vi "GetTestResult.vi"(11 "GuiRef":T1={"StringOut"=refnum, "AbortOnFail"=refnum, "SN"=refnum, "SN_Length"=refnum, "TestResult"=refnum, "CycleTime"=refnum, "ErrorCode"=refnum, "UUTStatus"=refnum, "DataBaseEnable?"=refnum, "DUTModel"=refnum, "FixtureID"=refnum, "OperatorID"=refnum, "SNReady"=refnum, "StopSlot"=refnum, "NextStep"=refnum, "PassYeild"=refnum, "Failed"=refnum, "Passed"=refnum, "Tested"=refnum, "TestItemsCtl"={"StepName"="", "TestEnable"=FALSE, "LoopCount"=0, "StopOnFail"=FALSE, "Index"=0, "TestName"="", "通道"="", "参数"="", "TimeStart"=0}, "ProcessBar"=refnum, "Slot"=enum."Slot1", "Row"=3, "States"=refnum, "TestMode"=refnum, "循环次数-DUT"=refnum, "波形图"=refnum, "产品型号"=refnum, "子面板"=refnum, "测试失败项目"=refnum, "测试结果"=refnum, "DUT"=refnum, "Starttime"=refnum, "SlotReady"=refnum, "版本信息"=refnum, "WIFI_1"=refnum, "WIFI_2"=refnum, "直通率"=refnum, "卡1开卡结果"=refnum, "卡2开卡结果"=refnum}) -> (1 "FailStep":string, 2 "PASS/FAIL":bool)   [LabVIEW 2013]
uses:
  SysControl/Reference.ctl
  SysControl/TestItemsCTL.ctl
  SysControl/Slot.ctl
  SysControl/LEDState.ctl
panel:
  out "FAIL项目":string
  out "PASS项目":string
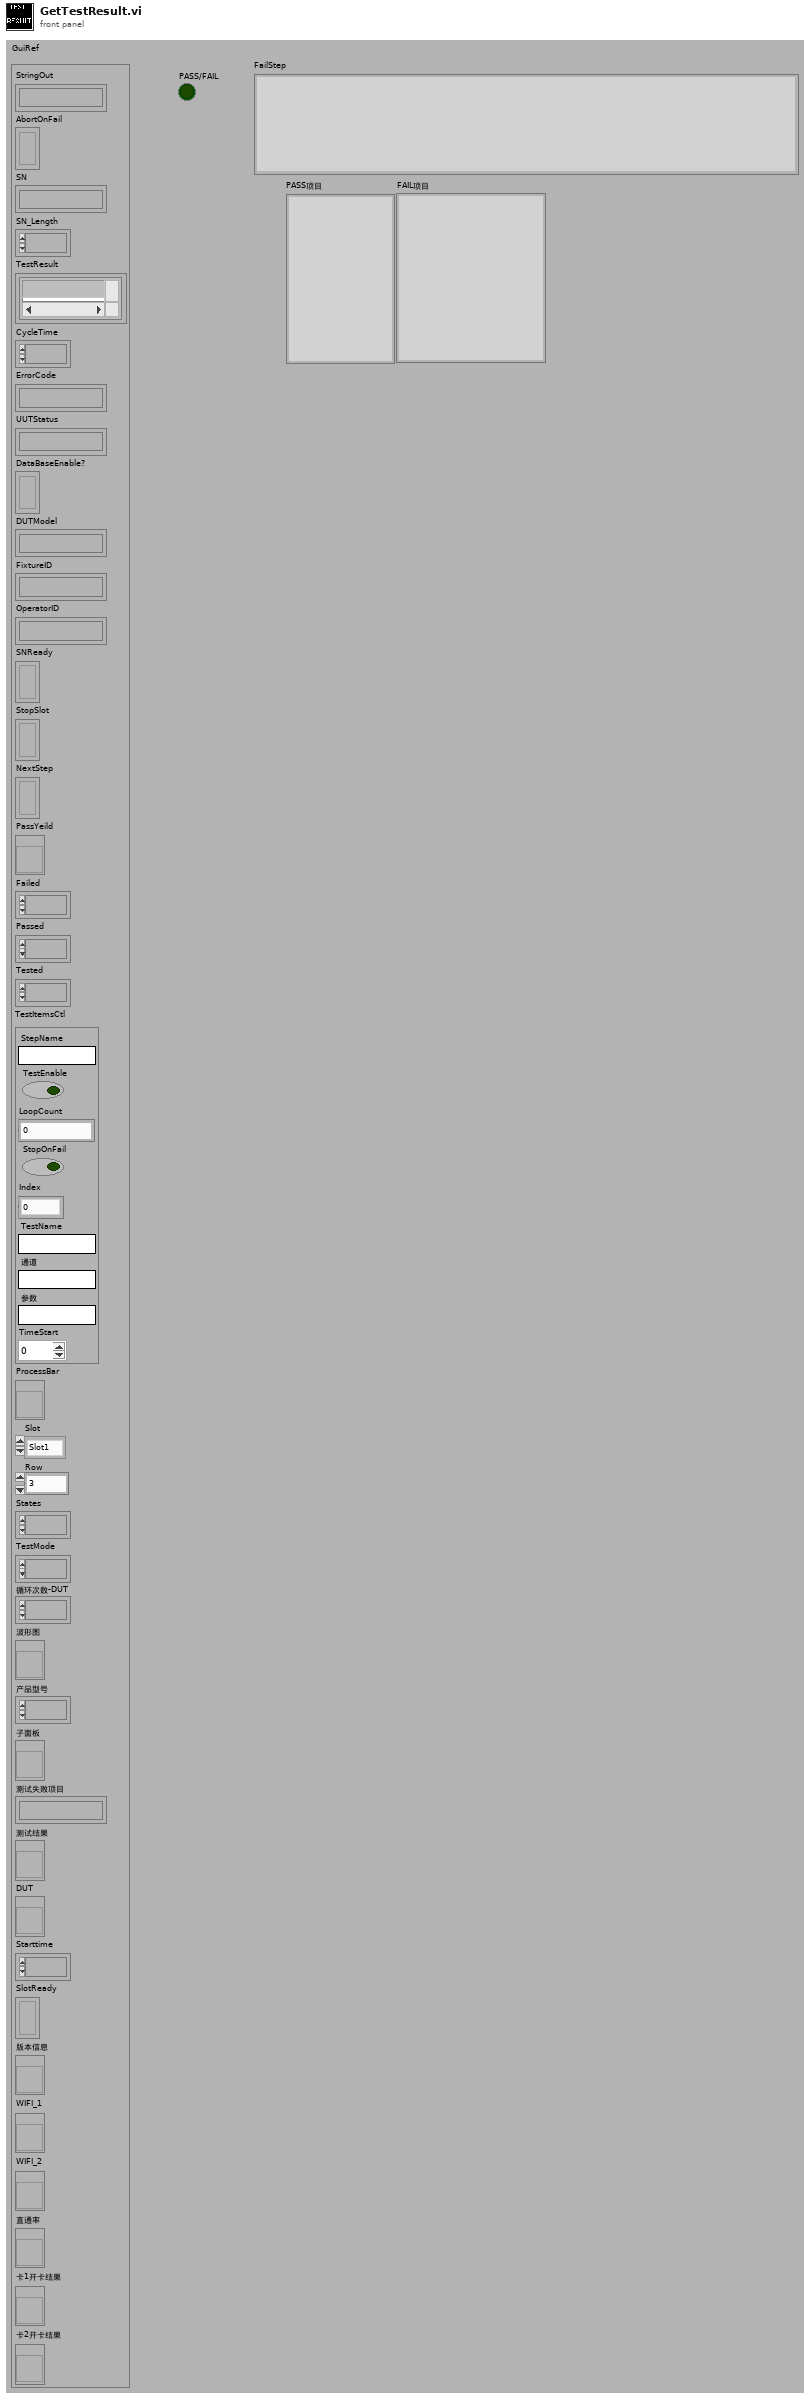
[diagram p1: front panel]
types:
  T1 = typedef "Reference.ctl" = cluster{"StringOut":refnum<vi>, "AbortOnFail":refnum<vi>, "SN":refnum<vi>, "SN_Length":refnum<vi>, "TestResult":refnum<vi>, "CycleTime":refnum<vi>, "ErrorCode":refnum<vi>, "UUTStatus":refnum<vi>, "DataBaseEnable?":refnum<vi>, "DUTModel":refnum<vi>, "FixtureID":refnum<vi>, "OperatorID":refnum<vi>, "SNReady":refnum<vi>, "StopSlot":refnum<vi>, "NextStep":refnum<vi>, "PassYeild":refnum<vi>, "Failed":refnum<vi>, "Passed":refnum<vi>, "Tested":refnum<vi>, "TestItemsCtl":T2, "ProcessBar":refnum<vi>, "Slot":T3, "Row":u32, "States":refnum<vi>, "TestMode":refnum<vi>, "循环次数-DUT":refnum<vi>, "波形图":refnum<vi>, "产品型号":refnum<vi>, "子面板":refnum<vi>, "测试失败项目":refnum<vi>, "测试结果":refnum<vi>, "DUT":refnum<vi>, "Starttime":refnum<vi>, "SlotReady":refnum<vi>, "版本信息":refnum<vi>, "WIFI_1":refnum<vi>, "WIFI_2":refnum<vi>, "直通率":refnum<vi>, "卡1开卡结果":refnum<vi>, "卡2开卡结果":refnum<vi>}
  T2 = typedef "TestItemsCTL.ctl" = cluster{"StepName":string, "TestEnable":bool, "LoopCount":i32, "StopOnFail":bool, "Index":u32, "TestName":string, "通道":string, "参数":string, "TimeStart":u32}
  T3 = typedef "Slot.ctl" = enum16{"Slot1", "Slot2", "Slot3", "Slot4"}
  T4 = typedef "LEDState.ctl" = enum16{"默认", "闪烁", "停止闪烁", "真", "假"}
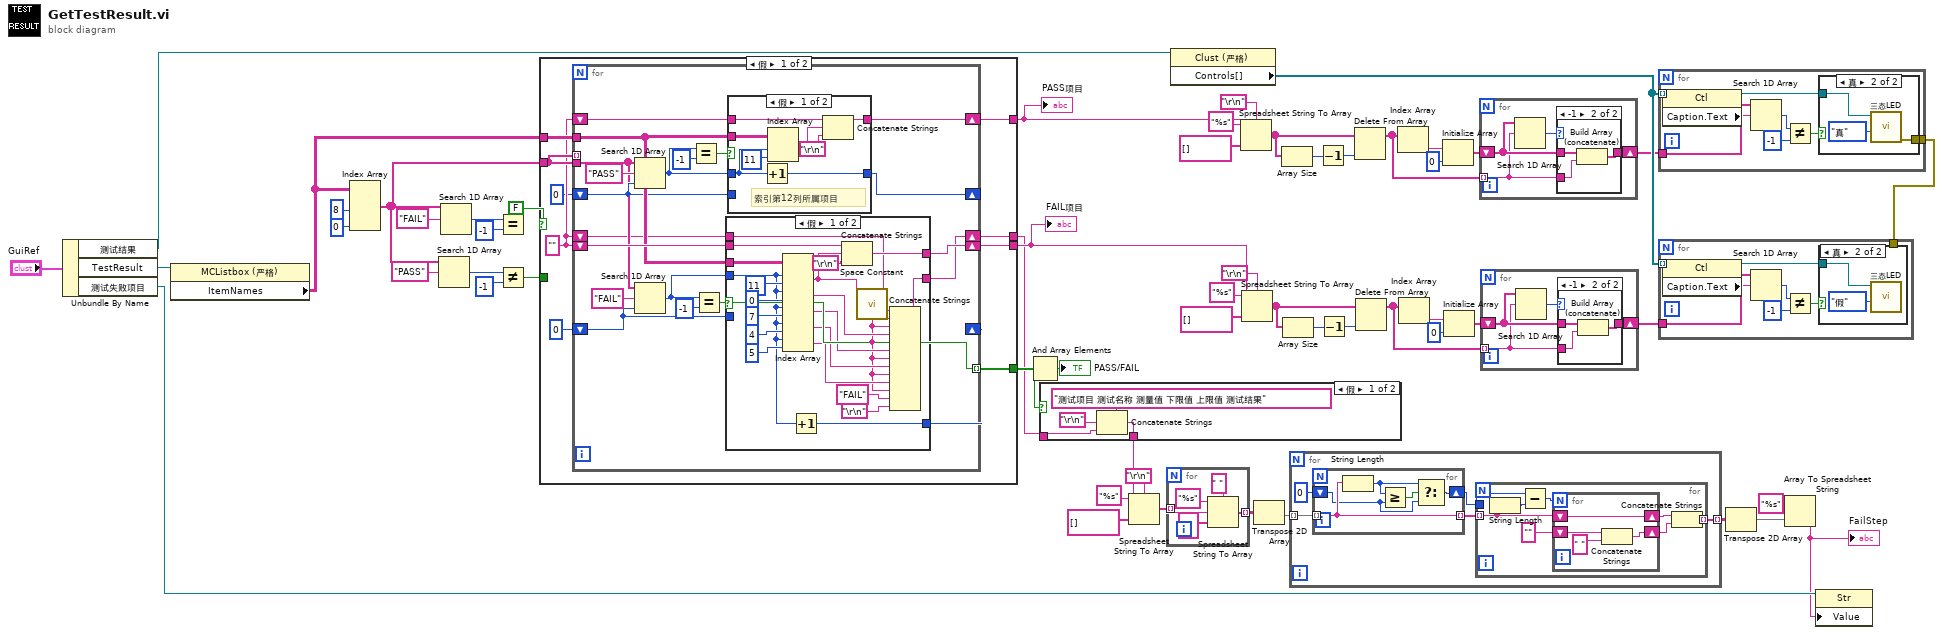
[diagram p0: block diagram]
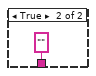
[diagram p2: hidden frame]
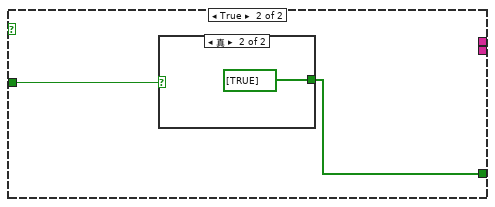
[diagram p9: hidden frame]
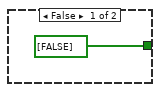
[diagram p10: hidden frame]
diagram:
  n1 = Unbundle By Name("GuiRef") -> ("测试结果"=w39:refnum<vi>, "TestResult"=w44:refnum<vi>, "测试失败项目"=w15:refnum<vi>)
  n2 = property class="MCListbox (严格)"(reference=w44) -> ("ItemNames"=w43:string[][])  [unwired: 1 in, 2 out]
  n3 = Index Array(array=w43, index (col) #1=8 ("禁用的索引 (列)"), index (col) #2=0 ("index (col)")) -> (element #1=w47:string[])  [unwired: 2 in, 1 out]
  n4 = Search 1D Array(1D array=w47, element="PASS" ("元素")) -> (index of element=w49:i32)  [unwired: 1 out]
  n5 = Search 1D Array(1D array=w47, element="FAIL" ("元素")) -> (index of element=w53:i32)  [unwired: 1 out]
  n6 = Equal?(x=w53, y=-1) -> ()  [unwired: 1 out]
  n7 = Not Equal?(x=w49, y=-1) -> (x != y?=w48:bool)
  n8 = case shown="假" FALSE {
    tunnel: w43 -> [w65 _]
    tunnel: w47 -> [w62 _]
    tunnel: [w64 w121] -> w52
    tunnel: [w63 _] -> w16
    tunnel: w48 -> [_ w120]
    tunnel: [w60 _] -> w19
    tunnel: [w58 _] -> w3
    frame False {
      w59 = "" ("字符串")
      n9 = for "For循环" {
        tunnel: w62 -> [w69]
        tunnel: w65 -> [w71]
        tunnel: [w81] -> w64 mode=indexing
        shift-right: [w72] -> w60
        shift-left: w59 -> [w73]
        shift-right: [w83] -> w63
        shift-left: w59 -> [w82]
        shift-right: [w79] -> _
        shift-left: 0 ("y") -> [w78]
        tunnel: w62 -> [_] mode=indexing
        shift-right: [w68] -> _
        shift-left: 0 -> [w70]
        shift-right: [w66] -> w58
        shift-left: w59 -> [w67]
        n10 = Search 1D Array(1D array=w69, element="PASS" ("元素"), start index (0)=w70) -> (index of element=w77:i32)
        n11 = Search 1D Array(1D array=w69, element="FAIL" ("元素"), start index (0)=w78) -> (index of element=w80:i32)
        n12 = Equal?(x=w77, y=-1) -> (x = y?=w76:bool)
        n13 = Equal?(x=w80, y=-1) -> (x = y?=w81:bool)
        n14 = case shown="假" w81 {
          tunnel: w71 -> [w115 _]
          tunnel: [w114 w119] -> w83
          tunnel: w82 -> [w113 w119]
          tunnel: w80 -> [w98 _]
          tunnel: [w112 w118] -> w79
          tunnel: w78 -> [_ w118]
          tunnel: w67 -> [w110 w117]
          tunnel: [w108 w117] -> w66
          frame False {
            n15 = Index Array(array=w115, index (row) #1=w98, index (col) #1=11 ("禁用的索引 (列)"), index (row) #2=w98, index (col) #2=0 ("禁用的索引 (列)"), index (row) #3=w98, index (col) #3=7 ("禁用的索引 (列)"), index (row) #4=w98, index (col) #4=4 ("禁用的索引 (列)"), index (row) #5=w98, index (col) #5=5 ("禁用的索引 (列)")) -> (element #1=w96:string, element #2=w99:string, element #3=w100:string, element #4=w101:string, element #5=w102:string)
            n16 = Increment(x=w98) -> (x+1=w112:i32)
            n17 = Concatenate Strings(w113, w96, "\r\n") -> (w114:string)
            n18 = call <vilib>:"Space Constant.vi"() -> ("String"=w97:string)
            n19 = Concatenate Strings(w110, w96, w97, w99, w97, w100, w97, w101, w97, w102, w97, "FAIL" ("字符串"), "\r\n") -> (w108:string)
          }
          frame True {
          }
        }
        n20 = case shown="假" w76 {
          tunnel: w71 -> [w92 _]
          tunnel: [w91 w95] -> w72
          tunnel: w73 -> [w90 w95]
          tunnel: w77 -> [w87 _]
          tunnel: [w88 w94] -> w68
          tunnel: w70 -> [_ w94]
          frame False {
            # "索引第12列所属项目"
            n21 = Increment(x=w87) -> (x+1=w88:i32)
            n22 = Index Array(array=w92, index (row)=w87, index (col)=11 ("禁用的索引 (列)")) -> (element=w89:string)
            n23 = Concatenate Strings(w90, w89, "\r\n") -> (w91:string)
          }
          frame True {
          }
        }
      }
    }
    frame True {
      n24 = case shown="真" w120 {
        tunnel: [bool[] [FALSE] bool[] [TRUE]] -> w121
        frame False {
        }
        frame True {
        }
      }
    }
  }
  "PASS项目" <- w19
  "FAIL项目" <- w16
  n25 = And Array Elements(Boolean array=w52) -> (logical AND=w2:bool)
  "PASS/FAIL" <- w2
  n26 = case shown="假" w2 {
    tunnel: [w126 ""] -> w4
    tunnel: w3 -> [w125 _]
    frame False {
      n27 = Concatenate Strings("测试项目 测试名称 测量值 下限值 上限值 测试结果" ("字符串"), "\r\n", w125) -> (w126:string)
    }
    frame True {
    }
  }
  n28 = Spreadsheet String To Array(delimiter (Tab)="\r\n", format string="%s" ("格式字符串"), spreadsheet string=w4, array type (2D Dbl)=string[] []) -> (array=w6:string[])
  n29 = for "For循环" {
    tunnel: w6 -> [w131] mode=indexing
    tunnel: [w129] -> w14 mode=indexing
    n30 = Spreadsheet String To Array(delimiter (Tab)=" " ("分隔符(Tab)"), format string="%s" ("格式字符串"), spreadsheet string=w131, array type (2D Dbl)=string[] []) -> (array=w129:string[])
  }
  n31 = property class="Clust (严格)"(reference=w39) -> ("Controls[]"=w30:refnum<vi>[])  [unwired: 1 in, 2 out]
  n32 = Spreadsheet String To Array(delimiter (Tab)="\r\n", format string="%s" ("格式字符串"), spreadsheet string=w19, array type (2D Dbl)=string[] []) -> (array=w29:string[])
  n33 = Spreadsheet String To Array(delimiter (Tab)="\r\n", format string="%s" ("格式字符串"), spreadsheet string=w16, array type (2D Dbl)=string[] []) -> (array=w32:string[])
  n34 = Transpose 2D Array(2D array=w14) -> (transposed array=w13:string[][])
  n35 = Array Size(array=w29) -> (size(s)=w26:i32)
  n36 = Array Size(array=w32) -> (size(s)=w35:i32)
  n37 = for "For循环" {
    tunnel: w13 -> [w136] mode=indexing
    tunnel: [w135] -> w10 mode=indexing
    n38 = for "For循环" {
      tunnel: w136 -> [w155] mode=indexing
      shift-right: [w151] -> w134
      shift-left: 0 -> [w153]
      tunnel: [w155] -> w137 mode=indexing
      n39 = String Length(string=w155) -> (length=w154:i32)
      n40 = Greater Or Equal?(x=w154, y=w153) -> (x >= y?=w152:bool)
      n41 = Select(t=w154, s=w152, f=w153) -> (s? t:f=w151:i32)
    }
    n42 = for "For循环" {
      tunnel: w137 -> [w139] mode=indexing
      tunnel: [w144] -> w135 mode=indexing
      tunnel: w134 -> [w142]
      n43 = String Length(string=w139) -> (length=w146:i32)
      n44 = Subtract(x=w142, y=w146) -> (x-y=w145:i32)
      n45 = for "For循环" {
        N: w145 -> [_]
        shift-right: [w148] -> w141
        shift-left: "" -> [w149]
        shift-right: [w147] -> w140
        shift-left: w139 -> [w147]
        n46 = Concatenate Strings(w149, " ") -> (w148:string)
      }
      n47 = Concatenate Strings(w140, w141) -> (w144:string)
    }
  }
  n48 = Decrement(x=w26) -> (x-1=w27:i32)
  n49 = Decrement(x=w35) -> (x-1=w34:i32)
  n50 = Delete From Array(array=w29, index=w27) -> (array with subset deleted=w28:string[])  [unwired: 1 in, 1 out]
  n51 = Delete From Array(array=w32, index=w34) -> (array with subset deleted=w33:string[])  [unwired: 1 in, 1 out]
  n52 = Index Array(array=w28) -> (element=w23:string)  [unwired: 1 in]
  n53 = Index Array(array=w33) -> (element=w38:string)  [unwired: 1 in]
  n54 = Initialize Array(w23, 0 ("维数大小")) -> (w25:string[])
  n55 = Initialize Array(w38, 0 ("维数大小")) -> (w36:string[])
  n56 = for "For循环" {
    shift-right: [w157] -> w18
    shift-left: w25 -> [w158]
    tunnel: w28 -> [w156] mode=indexing
    n57 = Search 1D Array(1D array=w158, element=w156) -> (index of element=w159:i32)  [unwired: 1 in]
    n58 = case shown="-1" w159 {
      tunnel: w158 -> [w160 w162]
      tunnel: [w160 w161] -> w157
      tunnel: w156 -> [_ w163]
      frame 1, Default {
      }
      frame -1 {
        n59 = Build Array (concatenate)(w162, w163) -> (w161:string[])
      }
    }
  }
  n60 = for "For循环" {
    shift-right: [w165] -> w31
    shift-left: w36 -> [w166]
    tunnel: w33 -> [w164] mode=indexing
    n61 = Search 1D Array(1D array=w166, element=w164) -> (index of element=w167:i32)  [unwired: 1 in]
    n62 = case shown="-1" w167 {
      tunnel: w166 -> [w168 w170]
      tunnel: [w168 w169] -> w165
      tunnel: w164 -> [_ w171]
      frame 1, Default {
      }
      frame -1 {
        n63 = Build Array (concatenate)(w170, w171) -> (w169:string[])
      }
    }
  }
  n64 = for "For循环" {
    tunnel: w30 -> [w179] mode=indexing
    tunnel: w18 -> [w178]
    tunnel: [w172] -> w17
    n65 = property class="Ctl"(reference=w179) -> (reference out=w173:refnum<vi>, "Caption.Text"=w177:string)  [unwired: 1 in, 1 out]
    n66 = Search 1D Array(1D array=w178, element=w177) -> (index of element=w176:i32)  [unwired: 1 in]
    n67 = Not Equal?(x=w176, y=-1) -> (x != y?=w174:bool)
    n68 = case shown="真" w174 {
      tunnel: w173 -> [_ w182]
      tunnel: [_ w180] -> w172
      frame False {
      }
      frame True {
        n69 = call "三态LED.vi"("State"=LEDState."真", "Ctl引用句柄"=w182) -> ("error out"=w180:errorcluster)  [unwired: 4 in, 1 out]
      }
    }
  }
  n70 = for "For循环" {
    tunnel: w30 -> [w189] mode=indexing
    tunnel: w31 -> [w188]
    tunnel: w17 -> [_]
    n71 = property class="Ctl"(reference=w189) -> (reference out=w183:refnum<vi>, "Caption.Text"=w187:string)  [unwired: 1 in, 1 out]
    n72 = Search 1D Array(1D array=w188, element=w187) -> (index of element=w186:i32)  [unwired: 1 in]
    n73 = Not Equal?(x=w186, y=-1) -> (x != y?=w184:bool)
    n74 = case shown="真" w184 {
      tunnel: w183 -> [_ w191]
      frame False {
      }
      frame True {
        n75 = call "三态LED.vi"("State"=LEDState."假", "Ctl引用句柄"=w191) -> ()  [unwired: 4 in, 2 out]
      }
    }
  }
  n76 = Transpose 2D Array(2D array=w10) -> (transposed array=w11:string[][])
  n77 = Array To Spreadsheet String(array=w11, 3:"%s" ("format string")) -> (spreadsheet string=w5:string)  [unwired: 1 out]
  "FailStep" <- w5
  n78 = property class="Str"(reference=w15, "Value"=w5) -> ()  [unwired: 1 in, 2 out]
